vi "Straight Line Equation.vi"() -> ()   [LabVIEW 2016]
panel:
  out "Y":dbl
  in  "Y-Intercept (b)":dbl
  in  "X":dbl
  in  "Slope (m)":dbl
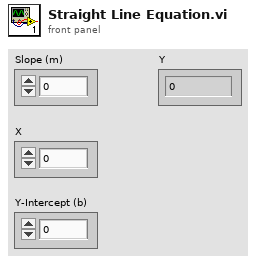
[diagram p1: front panel]
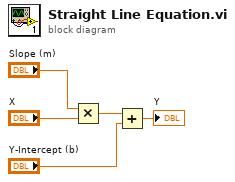
[diagram p0: block diagram]
diagram:
  n1 = Multiply(x="Slope (m)", y="X") -> (x*y=w3:dbl)
  n2 = Add(x=w3, y="Y-Intercept (b)") -> (x+y=→"Y":dbl)
